vi "Make_auxiliary_file.vi"(1 "Auxiliary Data":T1 {"EOS" items=["Ideal", "CH4_van_der_Waal", "CH4_Redlich_Kwong", "CO2_van_der_Waal", "CO2_Redlich_Kwong", ""]}, 2 "File Name":string) -> (0 "File Refnum":refnum<file>)   [LabVIEW 2016]
uses:
  auxiliary_cluster.ctl
  EOS.ctl
panel:
  in  "Error In":errorcluster
  out "Error Out":errorcluster
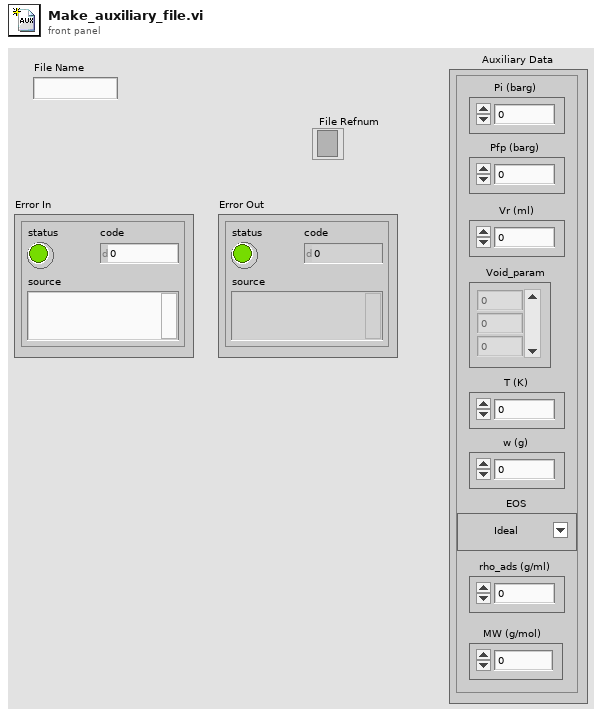
[diagram p1: front panel]
types:
  T1 = typedef "auxiliary_cluster.ctl" = cluster{"Pi (barg)":dbl, "Pfp (barg)":dbl, "Vr (ml)":dbl, "T (K)":dbl, "w (g)":dbl, "Void_param":dbl[], "EOS":T2, "rho_ads (g/ml)":dbl, "MW (g/mol)":dbl}
  T2 = typedef "EOS.ctl" = u16
  T3 = enum16{"open", "replace", "create", "open or create", "replace or create", "replace or create with confirmation"}
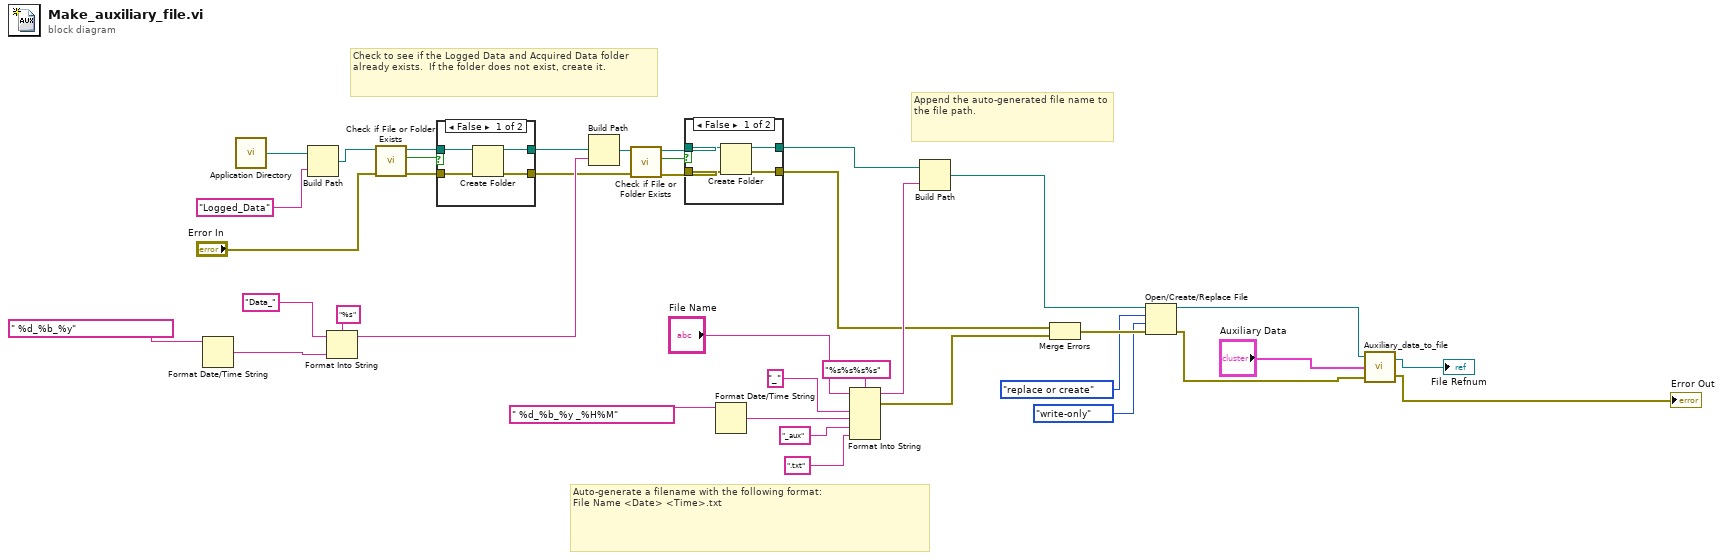
[diagram p0: block diagram]
diagram:
  # "Append the auto-generated file name to the file path."
  # "Check to see if the Logged Data and Acquired Data folder already exists.  If the folder does not exist, create it."
  # "Auto-generate a filename with the following format:\nFile Name <Date> <Time>.txt"
  n1 = Format Date/Time String(time format string (%c)=" %d_%b_%y") -> (date/time string=w20:string)  [unwired: 2 in]
  n2 = call <vilib>:"Application Directory.vi"() -> ("Application Directory"=w28:path)
  n3 = Build Path(base path=w28, name or relative path="Logged_Data" ("prompt (Create Folder)")) -> (appended path=w32:path)
  n4 = Format Into String(format string="%s", initial string="Data_" ("string"), w20) -> (resulting string=w18:string)  [unwired: 1 in, 1 out]
  n5 = call <vilib>:"Check if File or Folder Exists.vi"("error in (no error)"="Error In", "path"=w32) -> ("error out"=w31:errorcluster, "file or folder exists?"=w29:bool, "dup path"=w30:path)  [unwired: 7 in]
  n6 = case shown="False" w29 {
    tunnel: [w42 w44] -> w23
    tunnel: [w41 w43] -> w17
    tunnel: w31 -> [w40 w43]
    tunnel: w30 -> [w39 w44]
    frame False {
      n7 = Create Folder(path (use dialog)=w39, error in=w40) -> (created path=w42:path, error out=w41:errorcluster)  [unwired: 1 in, 1 out]
    }
    frame True {
    }
  }
  n8 = Build Path(base path=w23, name or relative path=w18) -> (appended path=w16:path)
  n9 = call <vilib>:"Check if File or Folder Exists.vi"("error in (no error)"=w17, "path"=w16) -> ("error out"=w13:errorcluster, "file or folder exists?"=w14:bool, "dup path"=w15:path)  [unwired: 7 in]
  n10 = case shown="False" w14 {
    tunnel: [w48 w50] -> w12
    tunnel: [w47 w49] -> w11
    tunnel: w13 -> [w46 w49]
    tunnel: w15 -> [w45 w50]
    frame False {
      n11 = Create Folder(path (use dialog)=w45, error in=w46) -> (created path=w48:path, error out=w47:errorcluster)  [unwired: 1 in, 1 out]
    }
    frame True {
    }
  }
  n12 = Format Date/Time String(time format string (%c)=" %d_%b_%y _%H%M") -> (date/time string=w9:string)  [unwired: 2 in]
  n13 = Format Into String(format string="%s%s%s%s", initial string="File Name", "_" ("input 1"), w9, "_aux" ("input 3"), ".txt" ("string")) -> (resulting string=w24:string, error out=w25:errorcluster)  [unwired: 1 in]
  n14 = Build Path(base path=w12, name or relative path=w24) -> (appended path=w38:path)
  n15 = Merge Errors(w11, w25) -> (w37:errorcluster)
  n16 = Open/Create/Replace File(file path (use dialog)=w38, error in=w37, operation (0:open)=T3."replace or create", access (0:read/write)=enum16{"read/write", "read-only", "write-only"}."write-only") -> (refnum out=w7:refnum<file>, error out=w5:errorcluster)  [unwired: 2 in, 1 out]
  n17 = call "Auxiliary_data_to_file.vi"("error in"=w5, "Auxiliary Data"="Auxiliary Data", "Byte Stream File in"=w7) -> ("error out"=→"Error Out":errorcluster, "Byte Stream File out"=→"File Refnum":refnum<file>)
